vi "ElevatorBump.vi"(1 "Elevator Goal In (in)":dbl) -> (0 "Elevator Goal Out (in)":dbl)   [LabVIEW 2018]
uses:
  Inputs_DriverStation.vi
panel:
  in  "Bump (in)":dbl=1.0
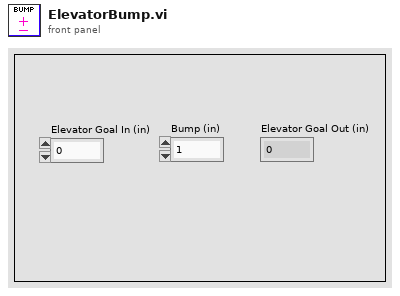
[diagram p1: front panel]
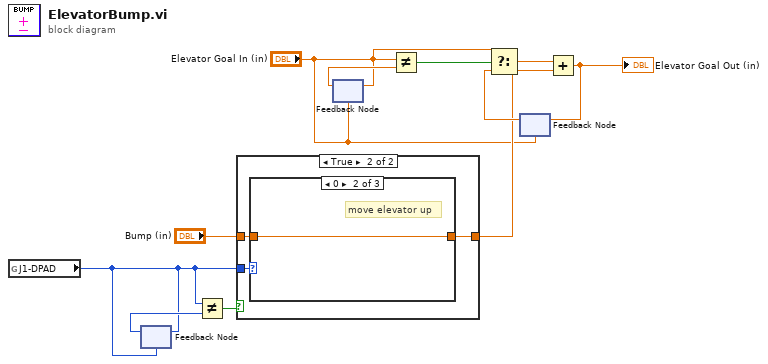
[diagram p0: block diagram]
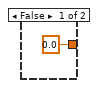
[diagram p2: hidden frame]
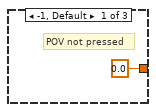
[diagram p3: hidden frame]
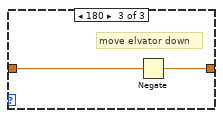
[diagram p4: hidden frame]
diagram:
  n1 = global read "Inputs_DriverStation.vi" "J1-DPAD"() -> (w1:i16)
  n2 = feedback-in #1(w1) -> ()
  n3 = feedback #1(w1) -> (w2:i16)
  n4 = Not Equal?(x=w1, y=w2) -> (x != y?=w3:bool)
  n5 = case shown="True" w3 {
    tunnel: w1 -> [_ w15]
    tunnel: "Bump (in)" -> [_ w14]
    tunnel: [0.0 ("Bump (in)") w13] -> w5
    frame False {
    }
    frame True {
      n6 = case shown="0" w15 {
        tunnel: [0.0 w17 w18] -> w13
        tunnel: w14 -> [_ w17 w19]
        frame -1, Default {
          # "POV not pressed"
        }
        frame 0 {
          # "move elevator up"
        }
        frame 180 {
          # "move elvator down"
          n7 = Negate(x=w19) -> (-x=w18:dbl)
        }
      }
    }
  }
  n8 = feedback-in #2("Elevator Goal In (in)") -> ()
  n9 = feedback #2("Elevator Goal In (in)") -> (w11:dbl)
  n10 = Not Equal?(x="Elevator Goal In (in)", y=w11) -> (x != y?=w10:bool)
  n11 = feedback #3("Elevator Goal In (in)") -> (w8:dbl)
  n12 = Select(t="Elevator Goal In (in)", s=w10, f=w8) -> (s? t:f=w9:dbl)
  n13 = Add(x=w9, y=w5) -> (x+y=w7:dbl)
  "Elevator Goal Out (in)" <- w7
  n14 = feedback-in #3(w7) -> ()
